vi "PLC.ReadPLCData.vi"(7 "Idx":i32, 8 "error in (no error)":errorcluster, 9 "Sets":T2, 10 "PLCdata in":T3, 11 "Ref in":u64) -> (0 "error out":errorcluster, 1 "Events":T1[](array[typedef]), 2 "PLCdata out":T3, 3 "Ref out":u64)   [LabVIEW 2016]
doc: "Read data block from PLC to PC, check live bit of PLC\n\nWabco 2017 All right reserved\nAuthor: maciej.szupienko@wabco-auto.com"
uses:
  PLC.DataBlock.PLCstatus.ctl
  PLC.DataBlock.PLCstatus.General.ctl
  PLC.DataBlock.PLCstatus.Station.ctl
  PLC.Data.Sets.ctl
  Tools/EventLog/EventLog.EventSource.ctl
  Tools/Translator/Translator.Message.ctl
  Tools/EventLog/EventLog.CreateError(array).vi
  Tools/EventLog/EventLog.New.vi
  Tools/EventLog/EventLog.New(array).vi
  Tools/ErrorHandling/ErrorHandling.Create.vi
  Global/ApplicationGlobal.vi
  Tools/EventLog/EventLog.Buffer.vi
  Tools/EventLog/EventLog.File.ReadWrite.vi
  Tools/Tma.lib/string.llb/Join array to string.vi
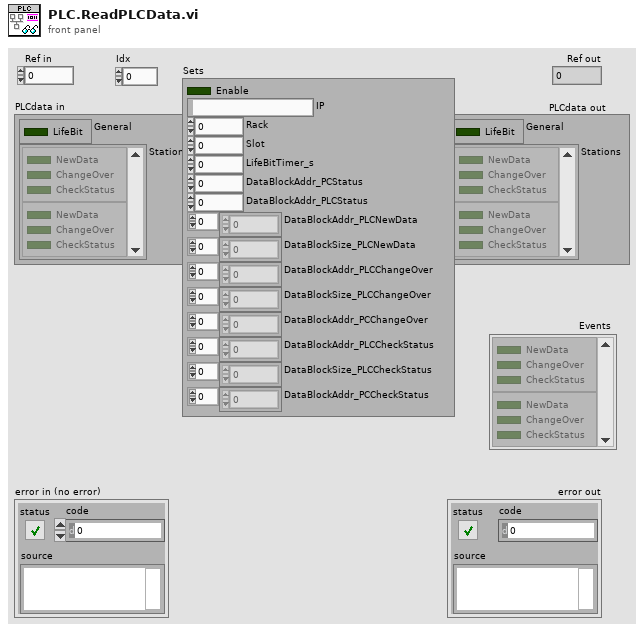
[diagram p1: front panel]
types:
  T1 = typedef "PLC.DataBlock.PLCstatus.Station.ctl" = cluster{"NewData":bool, "ChangeOver":bool, "CheckStatus":bool}
  T2 = typedef "PLC.Data.Sets.ctl" = cluster{"Enable":bool, "IP":string, "Rack":i32, "Slot":i32, "LifeBitTimer_s":dbl, "DataBlockAddr_PCStatus":i32, "DataBlockAddr_PLCStatus":i32, "DataBlockAddr_PLCNewData":i32[], "DataBlockSize_PLCNewData":i32[], "DataBlockAddr_PLCChangeOver":i32[], "DataBlockSize_PLCChangeOver":i32[], "DataBlockAddr_PCChangeOver":i32[], "DataBlockAddr_PLCCheckStatus":i32[], "DataBlockSize_PLCCheckStatus":i32[], "DataBlockAddr_PCCheckStatus":i32[]}
  T3 = typedef "PLC.DataBlock.PLCstatus.ctl" = cluster{"General":T4, "Stations":T1[]}
  T4 = typedef "PLC.DataBlock.PLCstatus.General.ctl" = cluster{"LifeBit":bool}
  T5 = typedef "Translator.Message.ctl" = enum16{"-", "Event confirmed", "Log out", "Log in", "Shutdown", "Cancel", "Start", "Continue", "Stop", "On", "Off", "OK", "NOK", "NOK %s", "This", "Prev", "Home", "Work", "In progress...", "Missing", "Empty", "Hardware failure", "Initial", "Error %d >> %s", "Error %d >> %s >> %s", "Starting %s", "Quitting %s", "Configured", "Initializing", "Quitting", "Loading", "Running %s", "Stopped", "Summary", "Do you want to continue?", "Do you want to exit?", "Log out?", "System", "All", "IDLE", "Translating...%s", "Not found", "Alarm %s", "Run", "Skip", "Abort", "Repeat", "Please wait...", "Database disconnected", "Login to database successful", "Login to database failed: %d; %s", "Get process step data for %s", "Changeover off", "Changeover into %s", "Product %s | %s found in cache with status %d at previous station", "Product %s | %s found in database with status %d at previous station", "Product %s | %s not found in cache at previous station", "Product %s | %s not found in database at previous station", "Product %s | %s found in cache with status %d at this station (%d repetion)", "Product %s | %s found in database with status %d at this station (%d repetition)", "Product %s | %s not found in cache at this station", "Product %s | %s not found in database at this station", "Product %s | %s found in cache for component %s | %s", "Product %s | %s found in database for component %s | %s", "Product not found in cache for component %s | %s", "Product not found in database for component %s | %s", "Product %s | %s connected with component %s | %s (cache)", "Product %s | %s connected with component %s | %s (database)", "New data for %s | %s (cache)", "New data for %s | %s (database)", "File %s moved (cache)", "File %s deleted (cache)", "Msg %d >> %s", "PLC LifeBit Failure", "Reconnecting DB", "Reconnecting PLC", "Free disk space is below 1GB - contact technician"}
  T6 = typedef "EventLog.EventSource.ctl" = enum16{"All", "Gui", "Cache", "PLC1", "PLC2", "PLC3", "DB", "DB01", "DB02", "DB03", "DB04", "DB05", "DB06", "DB07", "DB08", "DB09", "DB10", "DB11", "DB12", "DB13", "DB14", "DB15", "DB16"}
  T7 = cluster{"Boolean array[0]":bool, "Boolean array[1]":bool, "Boolean array[2]":bool, "Boolean array[3]":bool, "Boolean array[4]":bool, "Boolean array[5]":bool, "Boolean array[6]":bool, "Boolean array[7]":bool}
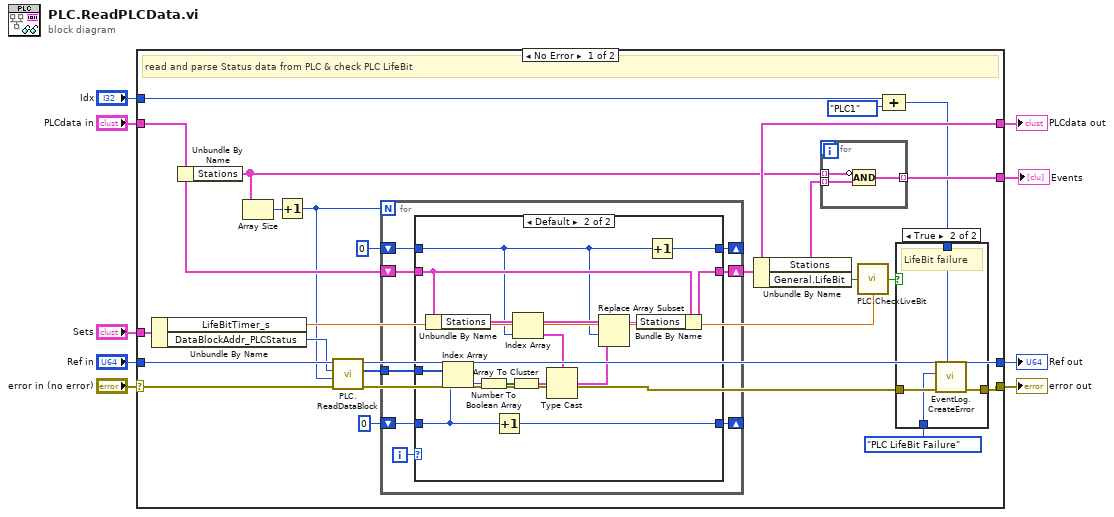
[diagram p0: block diagram]
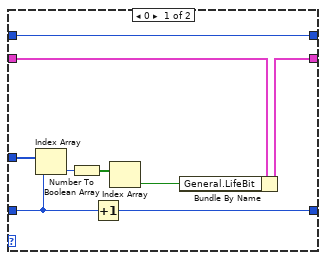
[diagram p2: hidden frame]
diagram:
  n1 = case shown="No Error" "error in (no error)" {
    selector: "error in (no error)" -> [w31 w75]
    tunnel: "Ref in" -> [w33 w74]
    tunnel: [w26 w75] -> w8
    tunnel: "PLCdata in" -> [w22 w73]
    tunnel: [w20 w73] -> w6
    tunnel: [w32 w74] -> w5
    tunnel: "Sets" -> [w30 _]
    tunnel: [w19 _] -> w1
    tunnel: "Idx" -> [w14 _]
    frame No Error {
      # "read and parse Status data from PLC & check PLC LifeBit"
      n2 = Unbundle By Name(w30) -> ("LifeBitTimer_s"=w25:dbl, "DataBlockAddr_PLCStatus"=w29:i32)
      n3 = Unbundle By Name(w22) -> ("Stations"=w18:T1[])
      n4 = Array Size(array=w18) -> (size(s)=w16:i32)
      n5 = Increment(x=w16) -> (x+1=w15:i32)
      n6 = call "PLC.ReadDataBlock.vi"("error in (no error)"=w31, "Amount (1)"=w15, "Block"=w29, "Ref"=w33) -> ("error out"=w27:errorcluster, "data out"=w24:u8[], "ref out"=w32:u64)  [unwired: 5 in]
      n7 = for {
        N: w15 -> [_]
        tunnel: w24 -> [w36]
        shift-right: [w39] -> _
        shift-left: 0 -> [w40]
        shift-right: [w37] -> w20
        shift-left: w22 -> [w38]
        shift-right: [w34] -> _
        shift-left: 0 -> [w35]
        i -> [w41]
        n8 = case shown="Default" w41 {
          tunnel: w40 -> [w43 w51]
          tunnel: [w47 w61] -> w39
          tunnel: w38 -> [w50 w60]
          tunnel: [w46 w63] -> w37
          tunnel: w36 -> [w49 w64]
          tunnel: w35 -> [w42 w52]
          tunnel: [w42 w53] -> w34
          frame 0 {
            n9 = Index Array(array=w49, index=w43) -> (element=w48:u8)
            n10 = Number To Boolean Array(number=w48) -> (Boolean array=w45:bool[])
            n11 = Increment(x=w43) -> (x+1=w47:i32)
            n12 = Index Array(array=w45) -> (element=w44:bool)  [unwired: 1 in]
            n13 = Bundle By Name(cluster=w50, "General.LifeBit"=w44) -> (w46:T3)
          }
          frame Default {
            n14 = Unbundle By Name(w60) -> ("Stations"=w56:T1[])
            n15 = Index Array(array=w64, index=w51) -> (element=w62:u8)
            n16 = Number To Boolean Array(number=w62) -> (Boolean array=w58:bool[])
            n17 = Increment(x=w51) -> (x+1=w61:i32)
            n18 = Array To Cluster(array=w58) -> (cluster=w57:T7)
            n19 = Index Array(array=w56, index=w52) -> (element=w55:T1)
            n20 = Type Cast(type=w55, x=w57) -> (*(type *) &x=w54:T1)
            n21 = Replace Array Subset(array=w56, new element=w54, index=w52) -> (w59:T1[])
            n22 = Bundle By Name(cluster=w60, "Stations"=w59) -> (w63:T3)
            n23 = Increment(x=w52) -> (x+1=w53:i32)
          }
        }
      }
      n24 = Unbundle By Name(w20) -> ("Stations"=w17:T1[], "General.LifeBit"=w21:bool)
      n25 = for {
        tunnel: w18 -> [w66] mode=indexing
        tunnel: w17 -> [w65] mode=indexing
        tunnel: [w67] -> w19 mode=indexing
        n26 = Compound Arithmetic op=AND(invert w66, w65) -> (w67:T1)
      }
      n27 = call "PLC.CheckLiveBit.vi"("LifeBit"=w21, "Timer [s] (3)"=w25) -> ("LiveBitElapsed"=w28:bool)
      n28 = Compound Arithmetic op=ADD(w14, EventLog.EventSource."PLC1" ("Event source")) -> (w12:i32)
      n29 = case shown="True" w28 {
        tunnel: w27 -> [w68 w72]
        tunnel: [w68 w71] -> w26
        tunnel: w12 -> [_ w70]
        tunnel: Translator.Message."PLC LifeBit Failure" ("Msg") -> [_ w69]
        frame False {
        }
        frame True {
          # "LifeBit failure"
          n30 = call-poly "EventLog.CreateError.vi"("Source (All)"=w70, "error in"=w72, "Msg"=w69) -> ("error out"=w71:errorcluster)  [unwired: 7 in, 1 out]
        }
      }
    }
    frame Error {
    }
  }
  "PLCdata out" <- w6
  "error out" <- w8
  "Ref out" <- w5
  "Events" <- w1
